vi "Page_Source_Remove.vi"(4 "sourceInclusion":T1, 6 "ctlReferences":T2, 7 "Project Refnum":refnum<vi>, 8 "error in (no error)":errorcluster, 9 "bottomTree?":bool, 10 "disableSource":bool, 11 "AB_Source_Container in":refnum<class "AB_Source_Container.lvclass">) -> (0 "error out":errorcluster, 3 "AB_Source_Container out":refnum<class "AB_Source_Container.lvclass">)   [LabVIEW 2020, in "AB_Source_Container.lvclass"]
uses:
  <vilib>/AppBuilder/AB_Classes/Source/Container/AB_Source_Container.lvclass
  e:/builds/penguin/labview/branches/2020/dev/dist/vi.lib/AppBuilder/AB_Classes/Source/AB_Source.lvclass
  <resource>/Framework/Providers/Builds/AppBuilder/AB_UI_Page_Source_Files_References.ctl
  <vilib>/AppBuilder/AB_Source_Inclusion.ctl
  <vilib>/AppBuilder/AB_Classes/Source/AB_Source.lvclass
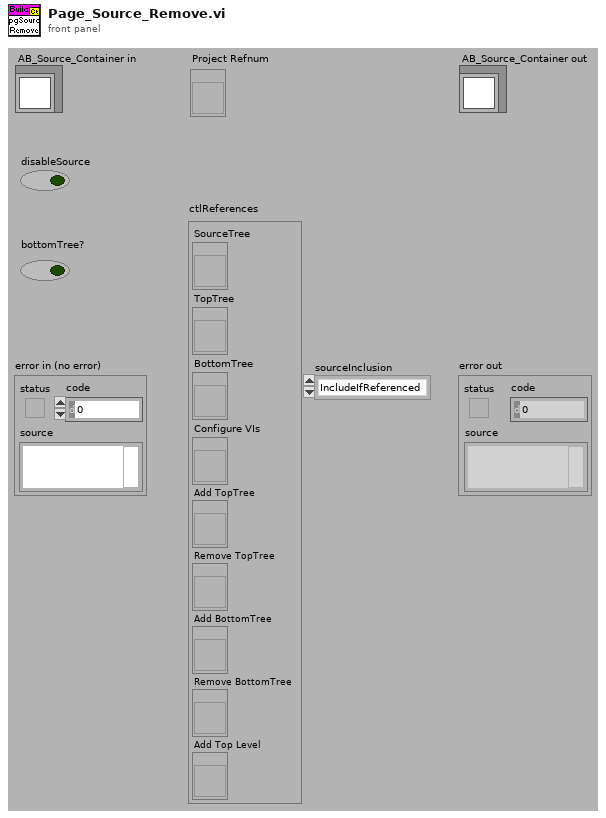
[diagram p1: front panel]
types:
  T1 = typedef "AB_Source_Inclusion.ctl" = enum16{"IncludeIfReferenced", "Include", "Exclude", "TopLevel"}
  T2 = typedef "AB_UI_Page_Source_Files_References.ctl" = cluster{"SourceTree":refnum<vi>, "TopTree":refnum<vi>, "BottomTree":refnum<vi>, "Configure VIs":refnum<vi>, "Add TopTree":refnum<vi>, "Remove TopTree":refnum<vi>, "Add BottomTree":refnum<vi>, "Remove BottomTree":refnum<vi>, "Add Top Level":refnum<vi>}
  T3 = typedef "AB_Source.ctl" = cluster{"path":path, "itemID":string, "parentIndex":i32, "sourceInclusion":T1, "destinationIndex":i32, "properties":T4[], "newName":string, "lvfile":bool, "valid":bool, "eng_inBuild":bool, "eng_isNonVILink":bool, "Amalgamation":bool, "Amalgamation Piece":bool, "eng_delimitedName":string, "preventRename":bool}
  T4 = typedef "AB_Source_Properties.ctl" = cluster{"sourcePropertyType":T5, "value":variant}
  T5 = typedef "AB_Source_Property_Type.ctl" = enum16{"Remove block diagram", "Remove front panel", "Password", "Window has title bar", "Show menu bar", "Show vertical scroll bar", "Show horizontal scroll bar", "Show toolbar", "Show Abort button", "Show fp when called", "Window behavior", "Allow user to close window", "Window run-time position", "Run when opened", "Allow debugging", "Auto error handling", "Generate guard code", "Use stack variables", "Expression folding", "Integer only", "Inline subVI"}
  T6 = typedef "AB_Source_Container.ctl" = cluster{"applyInclusion":bool, "applyDestination":bool, "applyProperties":bool, "applyPassword":bool, "applyPrefix":bool, "applySaveSetttings":bool, "dependentDestinationIndex":i32}
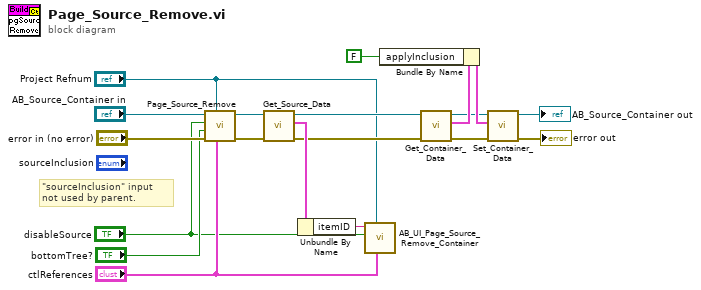
[diagram p0: block diagram]
diagram:
  # "\"sourceInclusion\" input not used by parent."
  n1 = call-parent "Page_Source_Remove.vi"("ctlReferences"="ctlReferences", "Project Refnum"="Project Refnum", "error in (no error)"="error in (no error)", "bottomTree?"="bottomTree?", "disableSource"="disableSource", "AB_Source in"="AB_Source_Container in") -> ("error out"=w8:errorcluster, "AB_Source out"=w10:refnum<class "AB_Source_Container.lvclass">)  [unwired: 4 in]
  n2 = call <vilib>:"Get_Source_Data.vi"("error in (no error)"=w8, "Class in"=w10) -> ("error out"=w7:errorcluster, "data"=w13:T3, "Class out"=w11:refnum<class "AB_Source_Container.lvclass">)  [unwired: 7 in]
  n3 = Unbundle By Name(w13) -> ("itemID"=w4:string)
  n4 = call <resource>:"AB_UI_Page_Source_Remove_Container.vi"("ctlReferences"="ctlReferences", "Project Refnum"="Project Refnum", "disableSource"="disableSource", "itemID"=w4) -> ()  [unwired: 7 in, 1 out]
  n5 = call <vilib>:"Get_Container_Data.vi"("error in (no error)"=w7, "Class in"=w11) -> ("error out"=w6:errorcluster, "data"=w16:T6, "Class out"=w12:refnum<class "AB_Source_Container.lvclass">)  [unwired: 7 in]
  n6 = Bundle By Name(cluster=w16, "applyInclusion"=FALSE) -> (w15:T6)
  n7 = call <vilib>:"Set_Container_Data.vi"("error in (no error)"=w6, "data"=w15, "Class in"=w12) -> ("error out"=→"error out":errorcluster, "Class out"=→"AB_Source_Container out":refnum<class "AB_Source_Container.lvclass">)  [unwired: 7 in]
